vi "Calculate Start and End Duty Cycle.vi"(10 "right annulus":T1={"Center X"=929, "Center Y"=663, "Inner Radius"=200, "Outer Radius"=405, "Start Angle"=90.0, "End Angle"=180.0} {"End Angle" format="%.2f"; "Start Angle" format="%.2f"; "Center X" scale=0.0..1024.0}, 11 "left annulus":T1={"Center X"=929, "Center Y"=663, "Inner Radius"=200, "Outer Radius"=405, "Start Angle"=90.0, "End Angle"=180.0} {"End Angle" format="%.2f"; "Start Angle" format="%.2f"; "Center X" scale=0.0..1024.0}) -> (0 "Right End Angle Duty Cycle":fxp<+,8,0>, 1 "Right Start Angle Duty Cycle":fxp<+,8,0>, 2 "Left End Angle Duty Cycle":fxp<+,8,0>, 3 "Left Start Angle Duty Cycle":fxp<+,8,0>)   [LabVIEW 2013]
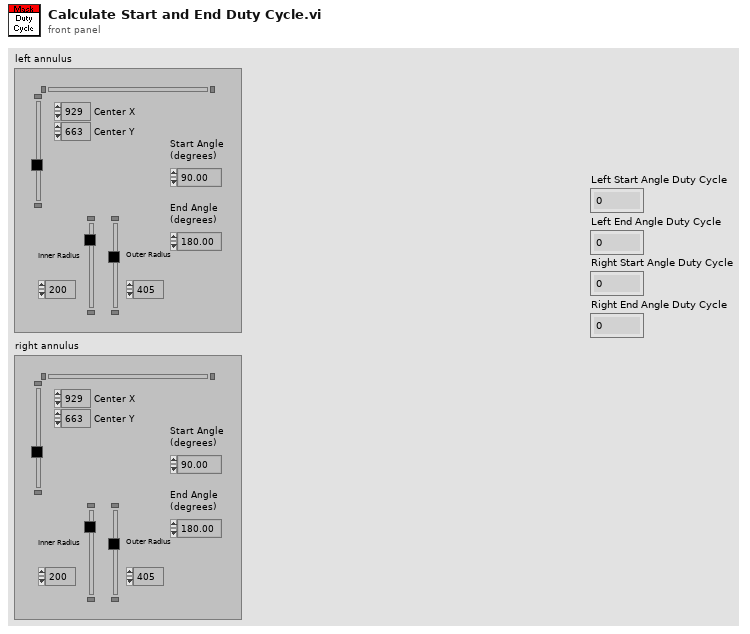
[diagram p1: front panel]
types:
  T1 = typedef "IMAQ Circle" = cluster{"Center X":i32, "Center Y":i32, "Inner Radius":i32, "Outer Radius":i32, "Start Angle":dbl, "End Angle":dbl}
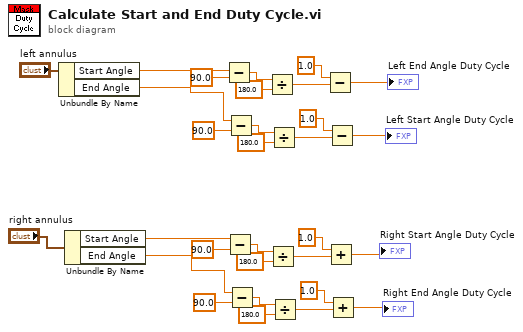
[diagram p0: block diagram]
diagram:
  n1 = Unbundle By Name("left annulus") -> ("Start Angle"=w28:dbl, "End Angle"=w16:dbl)
  n2 = Unbundle By Name("right annulus") -> ("Start Angle"=w4:dbl, "End Angle"=w3:dbl)
  n3 = Subtract(x=w28, y=90.0) -> (x-y=w26:dbl)
  n4 = Subtract(x=w4, y=90.0) -> (x-y=w6:dbl)
  n5 = Subtract(x=w16, y=90.0) -> (x-y=w18:dbl)
  n6 = Subtract(x=w3, y=90.0) -> (x-y=w13:dbl)
  n7 = Divide(x=w26, y=180.0) -> (x/y=w24:dbl)
  n8 = Divide(x=w6, y=180.0) -> (x/y=w8:dbl)
  n9 = Divide(x=w18, y=180.0) -> (x/y=w20:dbl)
  n10 = Divide(x=w13, y=180.0) -> (x/y=w11:dbl)
  n11 = Subtract(x=1.0, y=w24) -> (x-y=→"Left End Angle Duty Cycle":dbl)
  n12 = Add(x=1.0, y=w8) -> (x+y=→"Right Start Angle Duty Cycle":dbl)
  n13 = Subtract(x=1.0, y=w20) -> (x-y=→"Left Start Angle Duty Cycle":dbl)
  n14 = Add(x=1.0, y=w11) -> (x+y=→"Right End Angle Duty Cycle":dbl)
